vi "gyro.vi"   [LabVIEW 2013, in "mit2.lvrbt"]
uses:
  mit2.lvrbt
  <vilib>/NXT/Dual Mode Library/Sensors/EV3_Gyro_Rate.vi
  <vilib>/NXT/Dual Mode Library/Sensors/EV3_Gyro_Angle.vi
  <vilib>/NXT/Dual Mode Library/Waits/Wait_Num.vi
types:
  T1 = typedef "LVHSConnector.ctl" = refnum<class "BrickReference.lvclass">
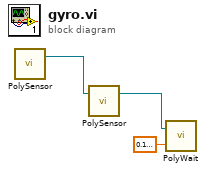
[diagram p0: block diagram]
diagram:
  n1 = call-poly <vilib>:"PolySensor.vi"() -> ("NXT/EV3"=w3:T1)  [unwired: 3 in, 1 out]
  n2 = call-poly <vilib>:"PolySensor.vi"("NXT/EV3"=w3) -> ("NXT/EV3"=w2:T1)  [unwired: 2 in, 1 out]
  n3 = call-poly <vilib>:"PolyWait.vi"("Time (1 sec)"=sgl 0.1, "NXT/EV3"=w2) -> ()  [unwired: 2 in, 1 out]
